vi "Ctor.vi"(8 "error in (no error)":errorcluster, 11 "Server Caching":T1) -> (0 "error out":errorcluster, 3 "Caching out":refnum<class "Caching.lvclass">)   [LabVIEW 2020, in "HTTP Server.lvlib" / "Caching.lvclass"]
uses:
  Caching.lvclass
  Server Caching.ctl
  Memory Cache.ctl
  Cache Item.ctl
  Caching.lvclass/Caching.ctl
  HTTP Server.lvlib
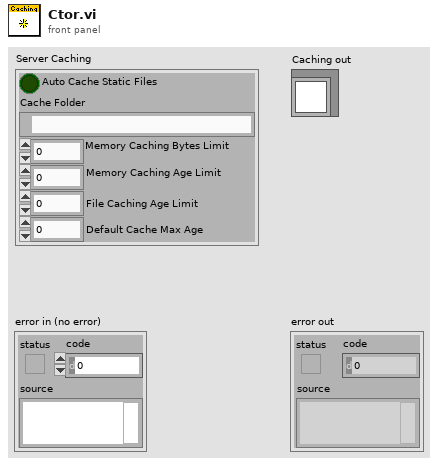
[diagram p1: front panel]
types:
  T1 = typedef "HTTP Server.lvlib/Server Caching.ctl" = cluster{"Auto Cache Static Files":bool, "Cache Folder":path, "Memory Caching Bytes Limit":i32, "Memory Caching Age Limit":dbl, "File Caching Age Limit":dbl, "Default Cache Max Age":i32}
  T2 = typedef "HTTP Server.lvlib/Caching.lvclass/Memory Cache.ctl" = cluster{"Size":i64, "Map":map{string, T3}}
  T3 = typedef "HTTP Server.lvlib/Caching.lvclass/Cache Item.ctl" = cluster{"ID":string, "File":bool, "Path":path, "Value":string, "Created":timestamp, "Expires":timestamp}
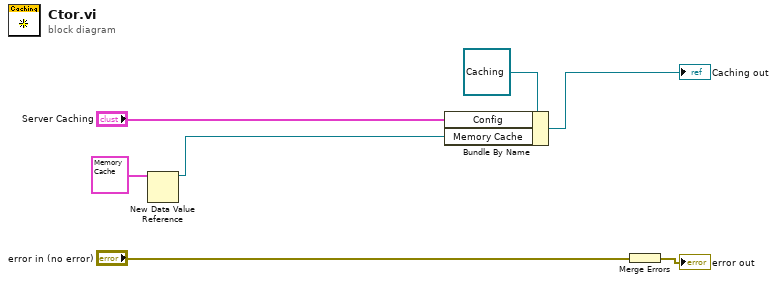
[diagram p0: block diagram]
diagram:
  n1 = New Data Value Reference(data value=T2 {"Size"=0, "Map"={}} ("Memory Cache")) -> (data value reference=w1:refnum<data-value>)  [unwired: 1 in, 1 out]
  n2 = Bundle By Name(cluster=refnum<class "Caching.lvclass"> refnum ("Caching in"), "Config"="Server Caching", "Memory Cache"=w1) -> (→"Caching out":refnum<class "Caching.lvclass">)
  n3 = Merge Errors("error in (no error)") -> (→"error out":errorcluster)
